vi "Thermal Chamber Response Simulator_Init-teardown.vi"(10 "Test Error":errorcluster, 11 "test case ID":string) -> (3 "result":bool)   [LabVIEW 2018]
doc: "The teardown VI should be executed after the VI under test in the harness VI. In this VI you can evaluate the outputs of the VI under test.\n\nSee the Help Document for more information. (<b>Help</b> > <b>IncQuery Labs</b> > <b>InstaCoverage</b> > <b>InstaCoverage Help...</b>)"
uses:
  Libraries/Thermal Chamber Response Simulator/Thermal Chamber Response Simulator.lvlib
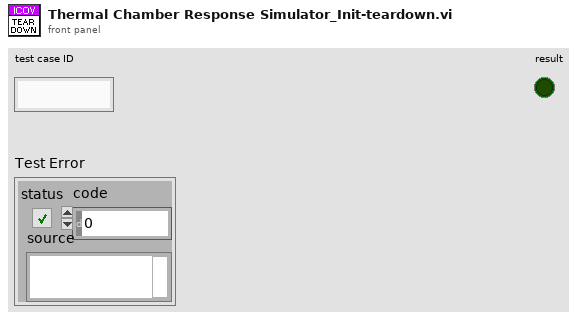
[diagram p1: front panel]
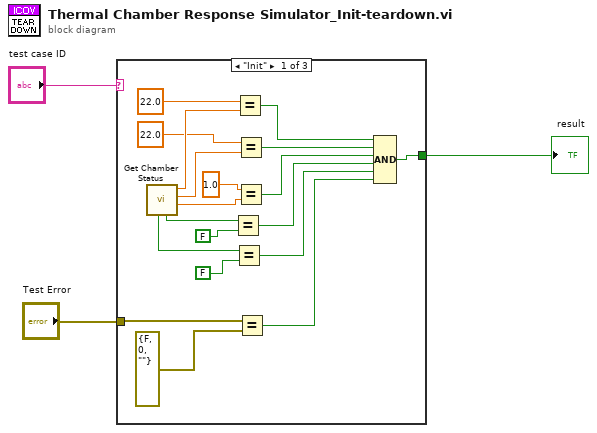
[diagram p0: block diagram]
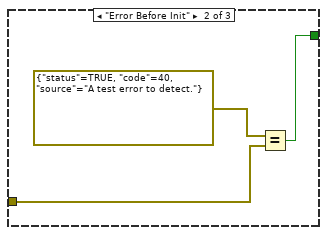
[diagram p2: hidden frame]
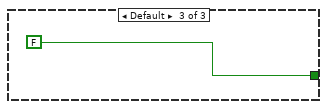
[diagram p3: hidden frame]
diagram:
  n1 = case shown="\"Init\"" "test case ID" {
    tunnel: [w7 w23 FALSE] -> w2
    tunnel: "Test Error" -> [w13 w24 _]
    frame "Init" {
      n2 = call "Get Chamber Status.vi"() -> ("Ramp Rate (deg C / second)"=w18:dbl, "Temperature Set Point (deg C)"=w16:dbl, "Actual Temperature"=w15:dbl, "Application Exit"=w21:bool, "Heater State"=w19:bool)  [unwired: 6 in, 1 out]
      n3 = Equal?(x=w21, y=FALSE) -> (x = y?=w8:bool)
      n4 = Equal?(x=w19, y=FALSE) -> (x = y?=w5:bool)
      n5 = Equal?(x=22.0, y=w15) -> (x = y?=w11:bool)
      n6 = Equal?(x=22.0, y=w16) -> (x = y?=w10:bool)
      n7 = Equal?(x=1.0, y=w18) -> (x = y?=w9:bool)
      n8 = Equal?(x=w13, y=errorcluster {"status"=FALSE, "code"=0, "source"=""} ("Test Error")) -> (x = y?=w6:bool)
      n9 = Compound Arithmetic op=AND(w11, w10, w9, w8, w5, w6) -> (w7:bool)
    }
    frame "Error Before Init" {
      n10 = Equal?(x=errorcluster {"status"=TRUE, "code"=40, "source"="A test error to detect."} ("error out"), y=w24) -> (x = y?=w23:bool)
    }
    frame Default {
    }
  }
  "result" <- w2
